vi "Lecroy_init.vi"(1 "Inst_parameters":T1={"Kind"=enum."LeCroy", "Strings"=["LeCroy", "192.168.137.1", "C1;C2", "V;V", "0;1", "1.0;1.0"], "uint64s"=[2, 12, 1, 0, 1, 4, 3], "Doubles"=[], "DAQmx take out list"=[]}) -> ()   [LabVIEW 2013]
uses:
  FPGA-clean_works_1.19f  - Matlab disabled/fpga-clean/host-subVIs/LeCroy Wave Series/LeCroy Wave Series.lvlib
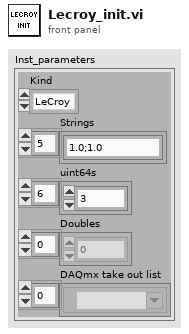
[diagram p1: front panel]
types:
  T1 = cluster{"Kind":enum16{"ADC", "K2000", "34401A", "LeCroy"}, "Strings":string[], "uint64s":u64[], "Doubles":dbl[], "DAQmx take out list":refnum<k21>[]}
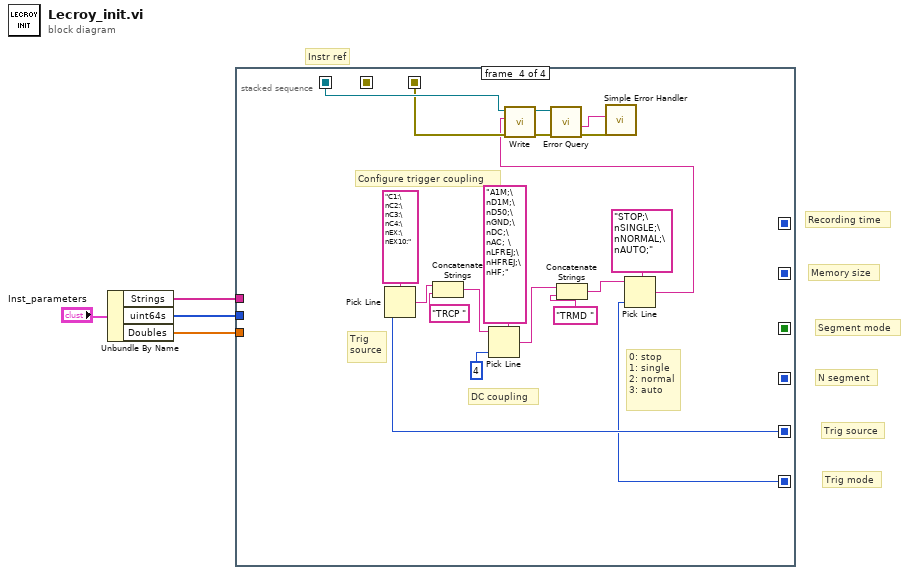
[diagram p0: block diagram]
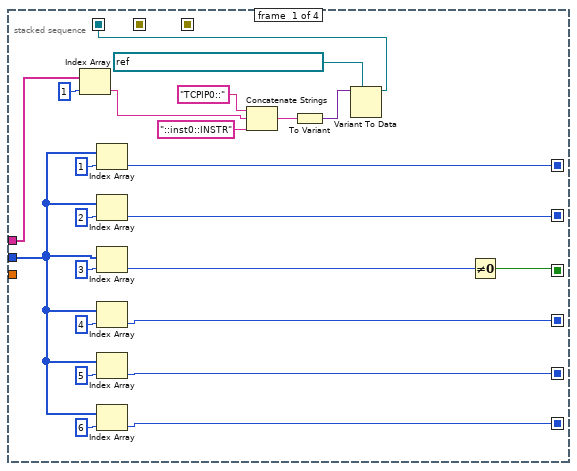
[diagram p2: hidden frame]
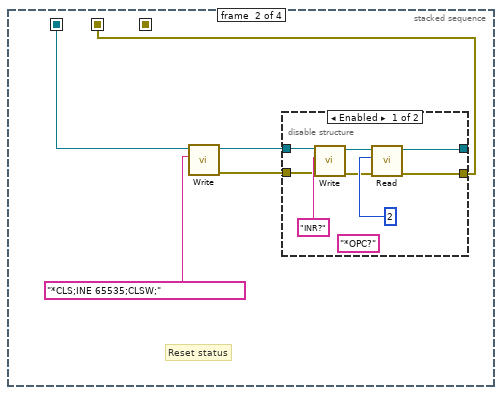
[diagram p3: hidden frame]
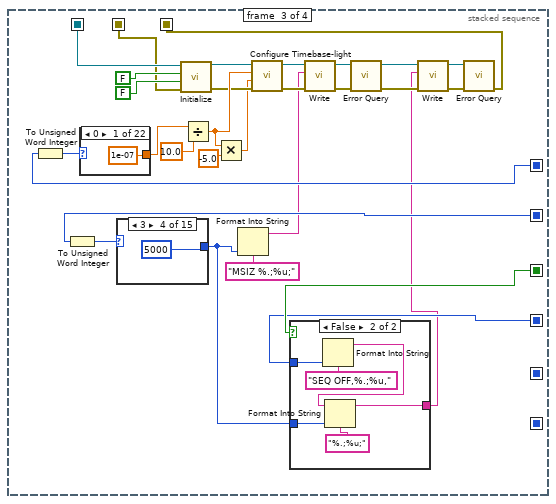
[diagram p5: hidden frame]
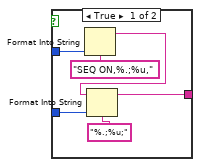
[diagram p6: hidden frame]
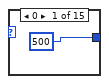
[diagram p7: hidden frame]
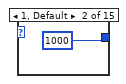
[diagram p8: hidden frame]
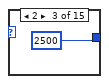
[diagram p9: hidden frame]
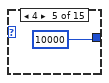
[diagram p10: hidden frame]
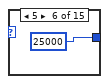
[diagram p11: hidden frame]
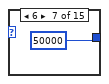
[diagram p12: hidden frame]
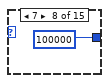
[diagram p13: hidden frame]
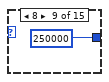
[diagram p14: hidden frame]
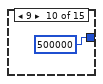
[diagram p15: hidden frame]
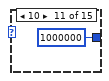
[diagram p16: hidden frame]
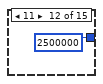
[diagram p17: hidden frame]
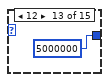
[diagram p18: hidden frame]
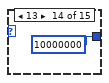
[diagram p19: hidden frame]
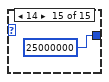
[diagram p20: hidden frame]
diagram:
  # "Trig mode"
  # "Trig source"
  # "N segment"
  # "Segment mode"
  # "Memory size"
  # "Recording time"
  # "Instr ref"
  n1 = Unbundle By Name("Inst_parameters") -> ("Strings"=w3:string[], "uint64s"=w2:u64[], "Doubles"=w1:dbl[])
  n2 = stacked-sequence {
    seq-local: [w19 _ _ _] -> [_ w29 w70 w126]
    seq-local: [w8 _ _ _] -> [_ _ w62 _]
    seq-local: [w7 _ _ _] -> [_ _ w58 _]
    seq-local: [w5 _ _ _] -> [_ _ w52 _]
    seq-local: [w9 _ _ _] -> [_ _ w50 _]
    seq-local: [w10 _ _ _] -> [_ _ _ w131]
    seq-local: [w11 _ _ _] -> [_ _ _ w129]
    seq-local: [_ w28 _ _] -> [_ _ w44 _]
    seq-local: [_ _ w43 _] -> [_ _ _ w125]
    tunnel: w3 -> [w27 _ _ _]
    tunnel: w2 -> [w12 _ _ _]
    tunnel: w1 -> [_ _ _ _]
    frame #0 {
      n3 = Index Array(array=w27, index=1) -> (element=w20:string)
      n4 = Index Array(array=w12, index=1) -> (element=w8:u64)
      n5 = Index Array(array=w12, index=2) -> (element=w7:u64)
      n6 = Index Array(array=w12, index=3) -> (element=w6:u64)
      n7 = Index Array(array=w12, index=4) -> (element=w9:u64)
      n8 = Index Array(array=w12, index=5) -> (element=w10:u64)
      n9 = Index Array(array=w12, index=6) -> (element=w11:u64)
      n10 = Concatenate Strings("TCPIP0::" ("string"), w20, "::inst0::INSTR" ("string")) -> (w25:string)
      n11 = To Variant(anything=w25) -> (Variant=w22:variant)
      n12 = Variant To Data(type=refnum<visa-resource-name> "TCPIP0::192.168.137.3::inst0::INSTR" ("VISA resource name"), Variant=w22) -> (data=w19:refnum<visa-resource-name>)  [unwired: 1 in, 1 out]
      n13 = Not Equal To 0?(x=w6) -> (x != 0?=w5:bool)
    }
    frame #1 {
      # "Reset status"
      n14 = call "Write.vi"("Write Buffer"="*CLS;INE 65535;CLSW;", "VISA resource name"=w29) -> ("error out"=w32:errorcluster, "VISA resource name out"=w31:refnum<visa-resource-name>)  [unwired: 1 in, 7 out]
      n15 = disable-structure shown="Enabled" {
        disable-tunnel: w32 -> [w37 w42]
        disable-tunnel: w31 -> [w36 w41]
        disable-tunnel: [w34 w42] -> w28
        disable-tunnel: [w33 w41] -> _
        frame Enabled {
          (unwired) "*OPC?" ("Write Buffer")
          n16 = call "Write.vi"("error in (no error)"=w37, "Write Buffer"="INR?", "VISA resource name"=w36) -> ("error out"=w35:errorcluster, "VISA resource name out"=w40:refnum<visa-resource-name>)  [unwired: 7 out]
          n17 = call "Read.vi"("error in (no error)"=w35, "Byte Count"=u32 2, "VISA resource name"=w40) -> ("error out"=w34:errorcluster, "VISA resource name out"=w33:refnum<visa-resource-name>)  [unwired: 7 out]
        }
        frame Disabled {
        }
      }
    }
    frame #2 {
      n18 = To Unsigned Word Integer(number=w62) -> (unsigned 16bit integer=w61:u16)
      n19 = To Unsigned Word Integer(number=w58) -> (unsigned 16bit integer=w59:u16)
      n20 = case shown="0" w61 {
        tunnel: [1e-07 2e-07 5e-07 1e-06 2e-06 5e-06 1e-05 2e-05 5e-05 0.0001 0.0002 0.0005 0.001 0.002 0.005 0.01 0.02 0.05 0.1 0.2 0.5 1.0] -> w69
        frame 0 {
        }
        frame 1 {
        }
        frame 2 {
        }
        frame 3 {
        }
        frame 4 {
        }
        frame 5 {
        }
        frame 6 {
        }
        frame 7 {
        }
        frame 8 {
        }
        frame 9 {
        }
        frame 10 {
        }
        frame 11 {
        }
        frame 12, Default {
        }
        frame 13 {
        }
        frame 14 {
        }
        frame 15 {
        }
        frame 16 {
        }
        frame 17 {
        }
        frame 18 {
        }
        frame 19 {
        }
        frame 20 {
        }
        frame 21 {
        }
      }
      n21 = case shown="3" w59 {
        tunnel: [u32 500 u32 1000 u32 2500 u32 5000 u32 10000 u32 25000 u32 50000 u32 100000 u32 250000 u32 500000 u32 1000000 u32 2500000 u32 5000000 u32 10000000 u32 25000000] -> w51
        frame 0 {
        }
        frame 1, Default {
        }
        frame 2 {
        }
        frame 3 {
        }
        frame 4 {
        }
        frame 5 {
        }
        frame 6 {
        }
        frame 7 {
        }
        frame 8 {
        }
        frame 9 {
        }
        frame 10 {
        }
        frame 11 {
        }
        frame 12 {
        }
        frame 13 {
        }
        frame 14 {
        }
      }
      n22 = call "Initialize.vi"("error in (no error)"=w44, "Reset? (T: Yes)"=FALSE, "ID Query? (T: Yes)"=FALSE, "VISA resource name"=w70) -> ("error out"=w64:errorcluster, "VISA resource name out"=w65:refnum<visa-resource-name>)  [unwired: 6 out]
      n23 = Divide(x=w69, y=10.0 ("x")) -> (x/y=w66:dbl)
      n24 = Multiply(x=w66, y=-5.0) -> (x*y=w63:dbl)
      n25 = Format Into String(format string="MSIZ %.;%u;", w51) -> (resulting string=w53:string)  [unwired: 2 in, 1 out]
      n26 = call "Configure Timebase-light.vi"("error in (no error)"=w64, "Position (0.0 s)"=w63, "Timebase (0.0005 s)"=w66, "VISA resource name"=w65) -> ("error out"=w54:errorcluster, "VISA resource name out"=w57:refnum<visa-resource-name>)  [unwired: 6 in]
      n27 = case shown="False" w52 {
        tunnel: w50 -> [w75 w81]
        tunnel: w51 -> [w74 w80]
        tunnel: [w73 w79] -> w45
        frame True {
          n28 = Format Into String(format string="SEQ ON,%.;%u,", w75) -> (resulting string=w78:string)  [unwired: 2 in, 1 out]
          n29 = Format Into String(format string="%.;%u;", initial string=w78, w74) -> (resulting string=w73:string)  [unwired: 1 in, 1 out]
        }
        frame False {
          n30 = Format Into String(format string="SEQ OFF,%.;%u,", w81) -> (resulting string=w84:string)  [unwired: 2 in, 1 out]
          n31 = Format Into String(format string="%.;%u;", initial string=w84, w80) -> (resulting string=w79:string)  [unwired: 1 in, 1 out]
        }
      }
      n32 = call "Write.vi"("error in (no error)"=w54, "Write Buffer"=w53, "VISA resource name"=w57) -> ("error out"=w55:errorcluster, "VISA resource name out"=w56:refnum<visa-resource-name>)  [unwired: 7 out]
      n33 = call "Error Query.vi"("error in (no error)"=w55, "VISA resource name"=w56) -> ("error out"=w46:errorcluster, "VISA resource name out"=w47:refnum<visa-resource-name>)  [unwired: 8 out]
      n34 = call "Write.vi"("error in (no error)"=w46, "Write Buffer"=w45, "VISA resource name"=w47) -> ("error out"=w48:errorcluster, "VISA resource name out"=w49:refnum<visa-resource-name>)  [unwired: 7 out]
      n35 = call "Error Query.vi"("error in (no error)"=w48, "VISA resource name"=w49) -> ("error out"=w43:errorcluster)  [unwired: 9 out]
    }
    frame #3 {
      # "Trig\nsource"
      # "DC coupling"
      # "Configure trigger coupling"
      # "0: stop\n1: single\n2: normal\n3: auto"
      n36 = Pick Line(multi-line string="C1:\nC2:\nC3:\nC4:\nEX:\nEX10:", line index=w131) -> (output string=w138:string)  [unwired: 1 out]
      n37 = Concatenate Strings(w138, "TRCP ") -> (w135:string)
      n38 = Pick Line(string ("")=w135, multi-line string="A1M;\nD1M;\nD50;\nGND;\nDC;\nAC; \nLFREJ;\nHFREJ;\nHF;", line index=u16 4) -> (output string=w133:string)
      n39 = Concatenate Strings(w133, "TRMD ") -> (w132:string)
      n40 = Pick Line(string ("")=w132, multi-line string="STOP;\nSINGLE;\nNORMAL;\nAUTO;", line index=w129) -> (output string=w124:string)
      n41 = call "Write.vi"("error in (no error)"=w125, "Write Buffer"=w124, "VISA resource name"=w126) -> ("error out"=w128:errorcluster, "VISA resource name out"=w127:refnum<visa-resource-name>)  [unwired: 7 out]
      n42 = call "Error Query.vi"("error in (no error)"=w128, "VISA resource name"=w127) -> ("error out"=w122:errorcluster, "Error Message"=w123:string)  [unwired: 8 out]
      n43 = call <vilib>:"Simple Error Handler.vi"("error source (\" \")"=w123, "error in (no error)"=w122) -> ()  [unwired: 3 in, 5 out]
    }
  }
